vi "Export Color Ramp to Clipboard.vi"(11 "ColorRamp in":refnum<vi>) -> ()   [LabVIEW 2021]
panel:
  in  "error in (no error)":errorcluster
  out "error out":errorcluster
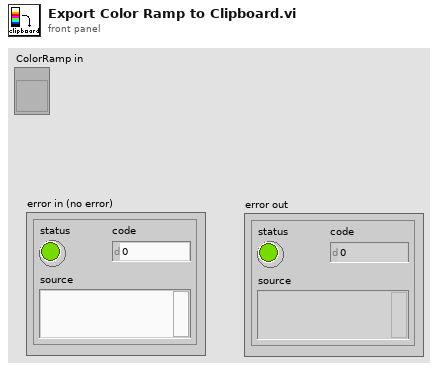
[diagram p1: front panel]
types:
  T1 = typedef "imagedata.ctl" = cluster{"image type":i32, "image depth":i32, "image":u8[], "mask":u8[], "colors":u32[], "Rectangle":cluster{"left":i16, "top":i16, "right":i16, "bottom":i16}}
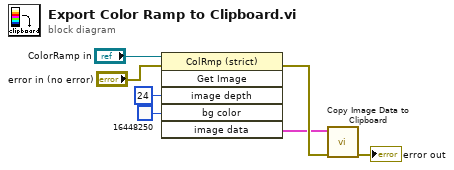
[diagram p0: block diagram]
diagram:
  n1 = invoke class="ColRmp (strict)" method="Get Image"(reference="ColorRamp in", error in="error in (no error)", "image depth"=24 ("Image Depth"), "bg color"=u32 16448250 ("Background Color")) -> (error out=w4:errorcluster, "image data"=w1:T1)  [unwired: 2 in, 4 out]
  n2 = call "Copy Image Data to Clipboard.vi"("error in (no error)"=w4, "image data"=w1) -> ("error out"=→"error out":errorcluster)  [unwired: 9 in]
